vi "sub_cal_flir.vi"(11 "FLIR cam data":i16[][](array[numeric])) -> (3 "temp data":dbl[][](array[numeric]))   [LabVIEW 2016]
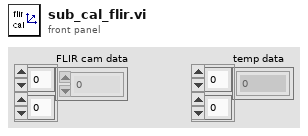
[diagram p1: front panel]
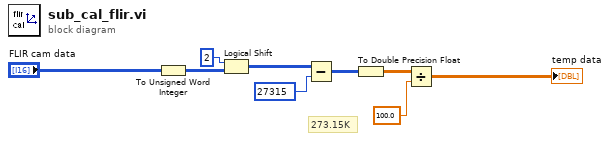
[diagram p0: block diagram]
diagram:
  # "273.15K"
  n1 = To Unsigned Word Integer(number="FLIR cam data") -> (unsigned 16bit integer=w6:u16[][])
  n2 = Logical Shift(y=i16 2, x=w6) -> (x << y=w2:u16[][])
  n3 = Subtract(x=w2, y=u16 27315) -> (x-y=w4:u16[][])
  n4 = To Double Precision Float(number=w4) -> (double precision float=w7:dbl[][])
  n5 = Divide(x=w7, y=100.0) -> (x/y=→"temp data":dbl[][])
